vi "Read Disable Auto Benchmark.vi"(8 "error in (no error)":errorcluster, 11 "CIFCorePlugin in":refnum<class "CIFCorePlugin.lvclass">) -> (0 "error out":errorcluster, 2 "Disable Auto Benchmark":bool, 3 "CIFCorePlugin out":refnum<class "CIFCorePlugin.lvclass">)   [LabVIEW 2021, in "CIFCorePlugin.lvclass"]
doc: "Disabling automatic benchmarking allows the user to control the benchmarking of the plugin manually. This is typically done if the logic loop may run multiple iterations per housekeeping cycle such as when external IO is rapidly being read. This is typically configured in the \"Create\" step. If automatic benchmarking is disabled the \"Benchmakr Execute\" function can be used to manually trigger benchmarking."
uses:
  CIFCorePlugin.lvclass
  CIFCorePlugin.lvclass/CIFCorePlugin.ctl
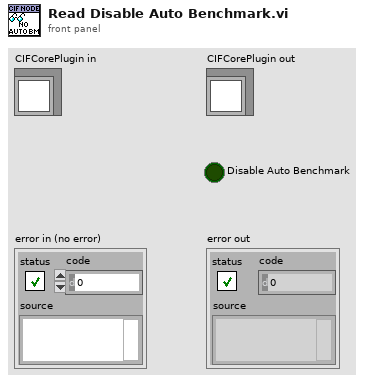
[diagram p1: front panel]
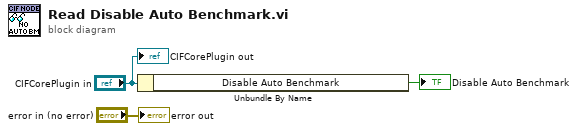
[diagram p0: block diagram]
diagram:
  n1 = Unbundle By Name("CIFCorePlugin in") -> ("Disable Auto Benchmark"=→"Disable Auto Benchmark":bool)
  "error out" <- "error in (no error)"
  "CIFCorePlugin out" <- "CIFCorePlugin in"
